vi "Main.vi"(11 "Module Admin":refnum<class "Delacor_lib_QMH_Module Admin.lvclass">) -> ()   [LabVIEW 2020, in "GetTemperature.lvlib"]
doc: "This template is based off of the Queued Message Handler design pattern and the Queued Message Handler project template that ships with LabVIEW.\n\nThe main difference is that the queue is private to this module and communication between modules is performed via Broadcast and Request events.\n\nRequest events are wrapped in public API methods and are handled in the Event Handling Loop (EHL) of this VI. Any module can register for Broadcast events sent by this module. The EHL generates messages based on user interface actions.\n\nThe Message Handling Loop (MHL) processes messages generated by the EHL, or by other messages. The messages are string values, so new messages can be added easily to the Message Cases case structure in the MHL. Each message cluster can also provide an optional value for Message Data, which is a variant that can be converted to whatever message-specific data is required.\n_____\nBased on Delacor QMH Project Template 4.0.0.47.\n_____\nBased on Delacor QMH Project Template 5.0.0.82."
uses:
  GetTemperature.lvlib
  <vilib>/Delacor/Delacor QMH/Libraries/Module Admin_class/Delacor_lib_QMH_Module Admin.lvclass
  Module Data--cluster.ctl
  Stop Argument--cluster.ctl
  <vilib>/Delacor/Delacor QMH/Libraries/Message Queue_class/Delacor_lib_QMH_Message Queue.lvclass/Delacor_lib_QMH_Message Queue.ctl
  <vilib>/Delacor/Delacor QMH/Libraries/Module Admin_class/Delacor_lib_QMH_Module Admin.lvclass/Delacor_lib_QMH_Module Admin.ctl
  Start Acquiring Argument--cluster.ctl
  Start Acquiring (Reply Payload)--cluster.ctl
  Stop Acquiring Argument--cluster.ctl
  Settings Editor/Update Application Settings (Reply Payload)--cluster.ctl
  Settings Editor/Settings--cluster.ctl
  <vilib>/Utility/miscctls.llb/LVPointTypeDef.ctl
  <vilib>/Delacor/Delacor QMH/Libraries/Message Queue_class/Delacor_lib_QMH_Enqueue Message (Single).vi
  <vilib>/Delacor/Delacor QMH/Libraries/Module Admin_class/Delacor_lib_QMH_Get External Launch.vi
  <vilib>/Utility/error.llb/Error Cluster From Error Code.vi
  <vilib>/ErrorRing/Error Ring.xnode
  <vilib>/Delacor/Delacor QMH/Libraries/Message Queue_class/Delacor_lib_QMH_Message Queue.lvclass
  Settings Editor/Settings Editor.lvlib
  Logger/FileLogging.lvlib
panel:
  out "Settings":T1 {"Units" items=["degC", "degF", "kelvin", "raw"]}
  out "Graph Data":waveform(dbl)[](array[waveform])
  out "error out":errorcluster
  # "This is a headless module. Show its panel to confirm that the Settings are updated correctly and other debugging tasks. Use the Settings Editor to change the settings for this module."
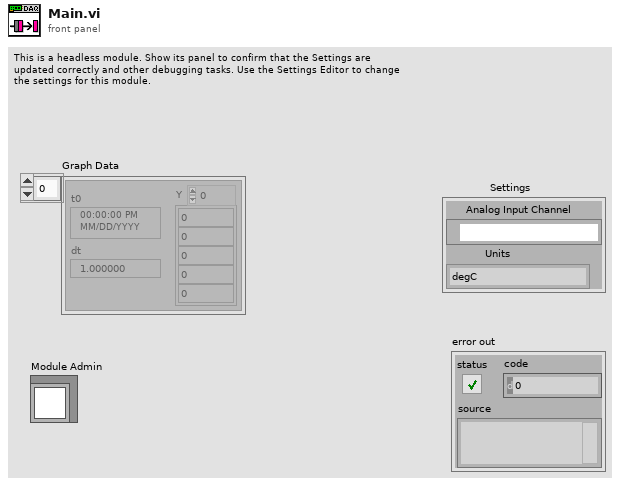
[diagram p1: front panel]
types:
  T1 = typedef "GetTemperature.lvlib/Module Data--cluster.ctl" = cluster{"Analog Input Channel":refnum<k21>, "Units":i32}
  T2 = typedef "Settings Editor.lvlib/Broadcast Events--cluster.ctl" = cluster{"Module Did Init":refnum<user-event>, "Status Updated":refnum<user-event>, "Error Reported":refnum<user-event>, "Module Did Stop":refnum<user-event>, "Update Module Execution Status":refnum<user-event>, "Application Settings Updated":refnum<user-event>}
  T3 = typedef "GetTemperature.lvlib/Request Events--cluster.ctl" = cluster{"Stop Module":refnum<user-event>, "Show Panel":refnum<user-event>, "Hide Panel":refnum<user-event>, "Get Module Execution Status":refnum<user-event>, "Show Diagram":refnum<user-event>, "Stop Acquiring":refnum<user-event>, "Wakeup Helper Loop":refnum<user-event>, "Change Settings":refnum<user-event>, "Calibrate DAQ":refnum<user-event>, "Start Acquiring":refnum<user-event>}
  T4 = enum32{"invalid lock state", "Not Locked", "Locked (No Password)", "Password-protected"}
  T5 = typedef "GetTemperature.lvlib/Stop Argument--cluster.ctl" = cluster{"Origin":string, "Exit via Stop Module Req?":bool, "Wait for Module to stop?":bool}
  T6 = typedef "GetTemperature.lvlib/Start Acquiring Argument--cluster.ctl" = cluster{"Wait Notifier":refnum<notifier>, "wait for reply":bool}
  T7 = typedef "GetTemperature.lvlib/Stop Acquiring Argument--cluster.ctl" = cluster{"Boolean":bool}
  T8 = typedef "Settings Editor.lvlib/Update Application Settings (Reply Payload)--cluster.ctl" = cluster{"Settings":T9, "Update Settings_error":errorcluster}
  T9 = typedef "Settings Editor.lvlib/Settings--cluster.ctl" = cluster{"Log File Base Path":path, "Analog Input Channel":refnum<k21>, "Units":i32}
  T10 = typedef "LVPointTypeDef.ctl" = cluster{"Horizontal":i16, "Vertical":i16}
  T11 = enum32{"Invalid", "Standard", "Closed", "Hidden", "Minimized", "Maximized"}
  T12 = typedef "GetTemperature.lvlib/Start Acquiring (Reply Payload)--cluster.ctl" = cluster{"HW ID":string, "Start Acquiring_error":errorcluster}
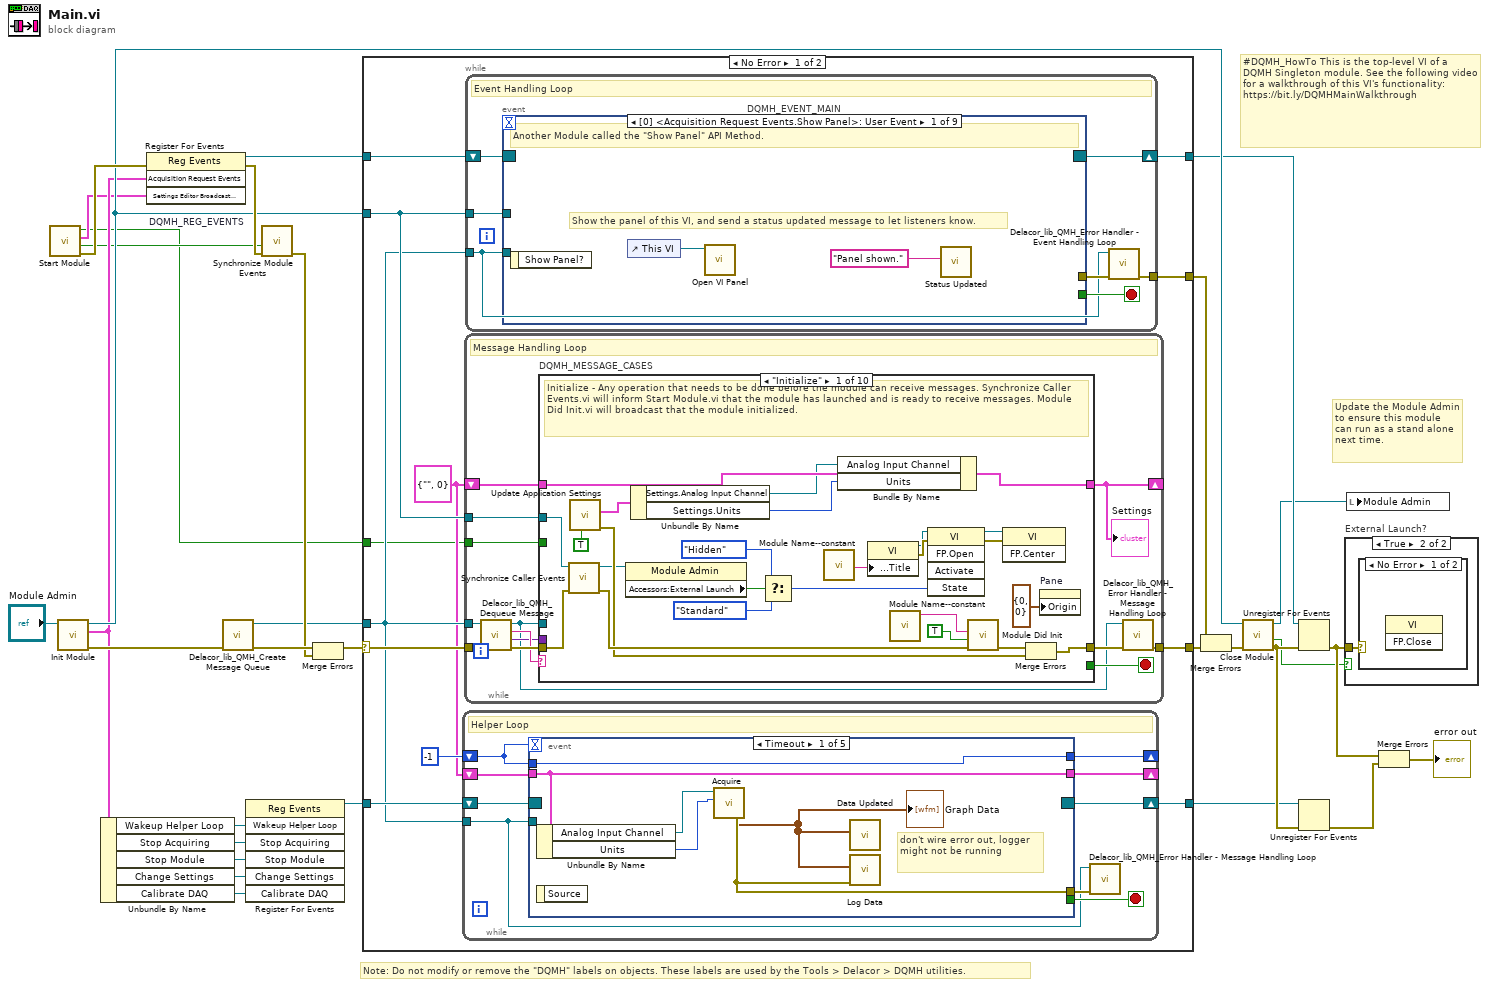
[diagram p0: block diagram]
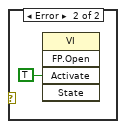
[diagram p3: hidden frame]
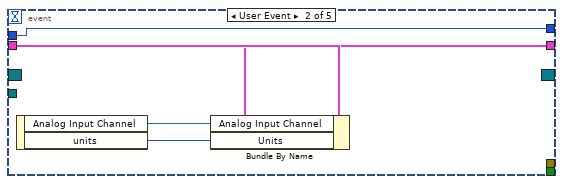
[diagram p4: hidden frame]
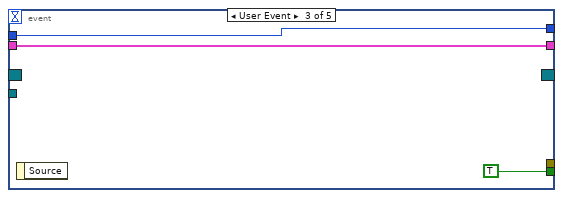
[diagram p5: hidden frame]
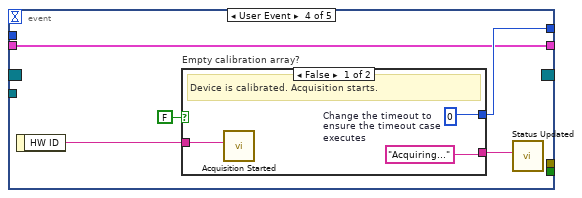
[diagram p6: hidden frame]
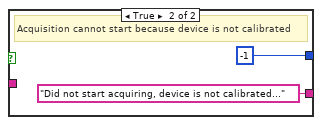
[diagram p7: hidden frame]
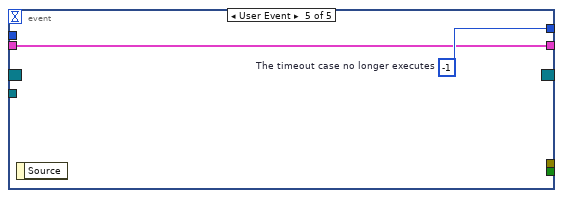
[diagram p8: hidden frame]
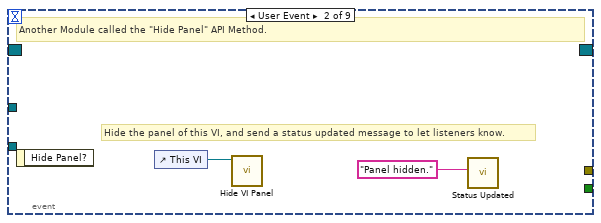
[diagram p9: hidden frame]
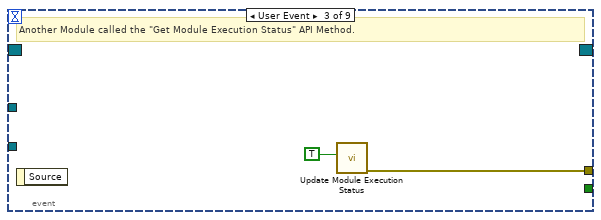
[diagram p10: hidden frame]
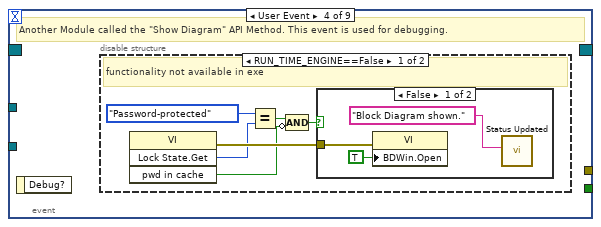
[diagram p11: hidden frame]
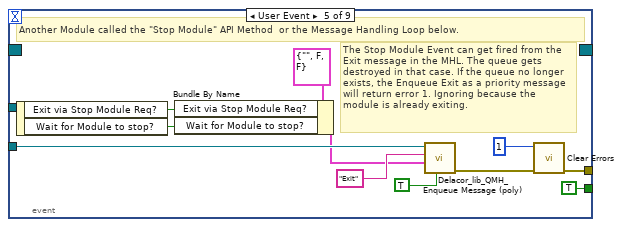
[diagram p14: hidden frame]
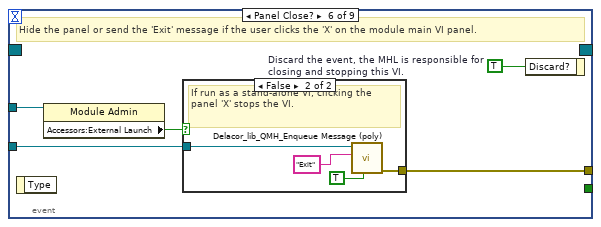
[diagram p15: hidden frame]
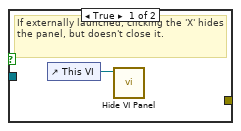
[diagram p16: hidden frame]
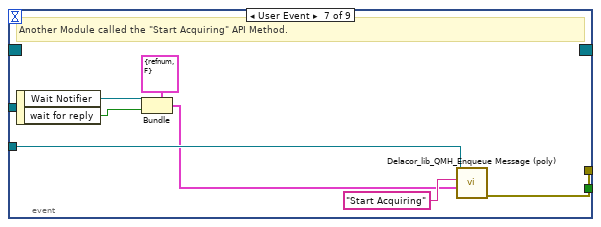
[diagram p17: hidden frame]
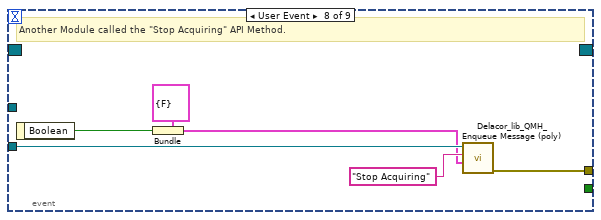
[diagram p18: hidden frame]
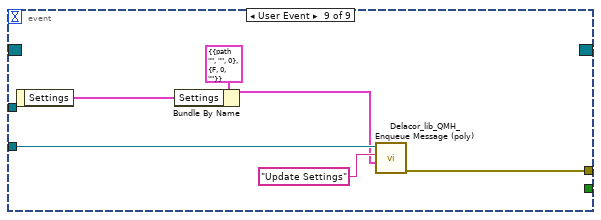
[diagram p19: hidden frame]
diagram:
  # "#DQMH_HowTo This is the top-level VI of a DQMH Singleton module. See the following video for a walkthrough of this VI's functionality: https://bit.ly/DQMHMainWalkthrough"
  # "Note: Do not modify or remove the \"DQMH\" labels on objects. These labels are used by the Tools > Delacor > DQMH utilities."
  # "Update the Module Admin to ensure this module can run as a stand alone next time."
  n1 = call "Start Module.vi"() -> ("error out"=w24:errorcluster, "Wait for Event Sync?"=w5:bool, "Settings Editor Broadcast Events"=w6:T2, "Module Was Already Running?"=w1:bool)  [unwired: 8 in]
  n2 = call "Init Module.vi"("Singleton Module Admin in"="Module Admin") -> ("error out"=w30:errorcluster, "Acquisition Request Events"=w11:T3, "Singleton Module Admin out"=w18:refnum<class "Delacor_lib_QMH_Module Admin.lvclass">)  [unwired: 8 in]
  n3 = Unbundle By Name(w11) -> ("Wakeup Helper Loop"=w7:refnum<user-event>, "Stop Acquiring"=w10:refnum<user-event>, "Stop Module"=w9:refnum<user-event>, "Change Settings"=w4:refnum<user-event>, "Calibrate DAQ"=w3:refnum<user-event>)
  n4 = register-events "DQMH_REG_EVENTS"(error in=w24, w11, w6) -> (reference out=w16:refnum<event-registration>, error out=w23:errorcluster)  [unwired: 1 in]
  n5 = call <vilib>:"Delacor_lib_QMH_Create Message Queue.vi"("error in (no error)"=w30) -> ("error out"=w26:errorcluster, "Message Queue"=w15:refnum<class "Delacor_lib_QMH_Message Queue.lvclass">)  [unwired: 9 in]
  n6 = register-events(w7, w10, w9, w4, w3) -> (reference out=w8:refnum<event-registration>)  [unwired: 2 in, 1 out]
  n7 = call "Synchronize Module Events.vi"("error in (no error)"=w23, "Wait for Event Sync?"=w5) -> ("error out"=w22:errorcluster)  [unwired: 9 in]
  n8 = Merge Errors(w26, w22) -> (w25:errorcluster)
  n9 = case shown="No Error" w25 {
    selector: w25 -> [w41 w274]
    tunnel: [w43 w273] -> w31
    tunnel: [w40 w282] -> w17
    tunnel: w16 -> [w39 w282]
    tunnel: w15 -> [w35 w275]
    tunnel: [w42 _] -> w29
    tunnel: w18 -> [w38 w278]
    tunnel: w8 -> [w36 w277]
    tunnel: [w33 w277] -> w2
    tunnel: w1 -> [w32 w276]
    frame No Error {
      w34 = T1 {"Analog Input Channel"="", "Units"=0} ("Data Cluster")
      n10 = while {
        shift-right: [w51] -> _
        shift-left: -1 -> [w50]
        tunnel: w35 -> [w47]
        shift-right: [w46] -> _
        shift-left: w34 -> [w45]
        shift-right: [w44] -> w33
        shift-left: w36 -> [w49]
        stop <- w48 stop-if-true
        # "Helper Loop"
        n11 = event shown="[0] Timeout" {
          selector: w49 -> [_ _ _ _ _]
          dyn-events: [_ _ _ _ _] -> w44
          timeout: w50 -> [_ _ _ _ _]
          tunnel: [w57 w63 w66 w71 w78] -> w51
          tunnel: w50 -> [w57 w63 w66 _ _]
          tunnel: [_ _ TRUE _ _] -> w48
          tunnel: w47 -> [_ _ _ _ _]
          tunnel: [w58 _ _ _ _] -> w52
          tunnel: [w56 w61 w64 w68 w77] -> w46
          tunnel: w45 -> [w56 w62 w64 w68 w77]
          event Timeout {
            # "don't wire error out, logger might not be running"
            n12 = Unbundle By Name(w56) -> ("Analog Input Channel"=w55:refnum<k21>, "Units"=w53:i32)
            n13 = event-data() -> ()  [unwired: 1 in, 1 out]
            n14 = call "Acquire.vi"("Units"=w53, "physical channels"=w55) -> ("error out"=w58:errorcluster, "Graph Data"=w54:waveform(dbl)[])  [unwired: 8 in]
            "Graph Data" <- w54
            n15 = call "Data Updated.vi"("Graph Data"=w54) -> ()  [unwired: 10 in, 1 out]
            n16 = call "Log Data.vi"("error in (no error)"=w58, "Waveforms"=w54) -> ()  [unwired: 9 in, 1 out]
          }
          event User Event {
            n17 = event-data() -> ("Analog Input Channel"=w60:refnum<k21>, "units"=w59:i32)  [unwired: 1 in]
            n18 = Bundle By Name(cluster=w62, "Analog Input Channel"=w60, "Units"=w59) -> (w61:T1)
          }
          event User Event {
            n19 = event-data() -> ()  [unwired: 1 in, 1 out]
          }
          event User Event {
            n20 = event-data() -> ("HW ID"=w69:string)  [unwired: 1 in]
            n21 = case "Empty calibration array?" shown="False" FALSE {
              tunnel: ["Acquiring..." ("Status") "Did not start acquiring, device is not calibrated..." ("Status")] -> w70
              tunnel: [w73 -1] -> w71
              tunnel: w69 -> [w74 _]
              frame False {
                w73 = 0  # Change the timeout to ensure the timeout case executes
                # "Device is calibrated. Acquisition starts."
                n22 = call "Acquisition Started.vi"("HW ID"=w74) -> ()  [unwired: 10 in, 1 out]
              }
              frame True {
                # "Acquisition cannot start because device is not calibrated"
              }
            }
            n23 = call "Status Updated.vi"("Status"=w70) -> ()  [unwired: 10 in, 1 out]
          }
          event User Event {
            w78 = -1  # The timeout case no longer executes
            n24 = event-data() -> ()  [unwired: 1 in, 1 out]
          }
        }
        n25 = call-dynamic "Delacor_lib_QMH_Error Handler - Message Handling Loop.vi"("error in (no error)"=w52, "Message Queue in"=w47) -> ()  [unwired: 8 in, 2 out]
      }
      n26 = while {
        tunnel: w35 -> [w145]
        shift-right: [w141] -> _
        shift-left: w34 -> [w149]
        tunnel: w41 -> [w152]
        tunnel: [w150] -> w43
        tunnel: w38 -> [w143]
        tunnel: w32 -> [w142]
        stop <- w148 stop-if-true
        # "Message Handling Loop"
        n27 = call-dynamic "Delacor_lib_QMH_Dequeue Message.vi"("error in (no error)"=w152, "Message Queue in"=w145) -> ("error out"=w151:errorcluster, "Message Data"=w146:variant, "Message"=w147:string, "Message Queue out"=w144:refnum<class "Delacor_lib_QMH_Message Queue.lvclass">)  [unwired: 6 in]
        n28 = case "DQMH_MESSAGE_CASES" shown="\"Initialize\"" w147 {
          selector: w147 -> [_ _ _ _ _ _ _ _ _ w260]
          tunnel: w144 -> [_ _ _ _ _ _ _ w225 w249 _]
          tunnel: w151 -> [w176 w180 w193 w207 w216 w219 w221 w232 w256 w263]
          tunnel: [w173 w180 w191 w205 w210 w218 w221 w228 w253 w264] -> w153
          tunnel: w149 -> [w163 w179 w181 w202 w213 w217 w220 w227 w241 w261]
          tunnel: [w158 w179 w189 w202 w213 w217 w220 w227 w241 w261] -> w141
          tunnel: [_ _ _ _ _ _ _ _ w248 _] -> w148
          tunnel: w146 -> [_ _ w188 w204 w214 _ _ w226 w247 _]
          tunnel: w143 -> [w164 _ _ _ _ _ _ w224 w242 _]
          tunnel: w142 -> [_ _ _ _ _ _ _ _ w239 _]
          frame "Initialize" {
            # "Initialize - Any operation that needs to be done before the module can receive messages. Synchronize Caller Events.vi will inform Start Module.vi that the module has launched and is ready to receive messages. Module Did Init.vi will broadcast that the module initialized."
            n29 = call "Synchronize Caller Events.vi"("error in (no error)"=w176, "Singleton Module Admin in"=w164) -> ("error out"=w175:errorcluster, "Singleton Module Admin out"=w160:refnum<class "Delacor_lib_QMH_Module Admin.lvclass">)  [unwired: 8 in]
            n30 = call "Update Application Settings.vi"("wait for reply (T)"=TRUE) -> ("error out"=w172:errorcluster, "Reply Payload"=w157:T8)  [unwired: 8 in, 1 out]
            n31 = property class="Module Admin"(reference=w160) -> ("Accessors:External Launch"=w168:bool)  [unwired: 1 in, 2 out]
            n32 = Unbundle By Name(w157) -> ("Settings.Analog Input Channel"=w155:refnum<k21>, "Settings.Units"=w154:i32)
            n33 = Select(t=T11."Hidden" ("State"), s=w168, f=T11."Standard" ("State")) -> (s? t:f=w165:T11)
            n34 = call "Module Name--constant.vi"() -> ("Module Name"=w171:string)  [unwired: 11 in]
            n35 = Bundle By Name(cluster=w163, "Analog Input Channel"=w155, "Units"=w154) -> (w158:T1)
            n36 = property class="VI"("Front Panel.Title"=w171) -> (reference out=w170:refnum<vi>, error out=w178:errorcluster)  [unwired: 2 in]
            n37 = call "Module Name--constant.vi"() -> ("Module Name"=w161:string)  [unwired: 11 in]
            n38 = invoke class="VI" method="FP.Open"(reference=w170, error in=w178, "State"=w165) -> (reference out=w169:refnum<vi>, error out=w177:errorcluster)  [unwired: 2 in, 3 out]
            n39 = call "Module Did Init.vi"("error in (no error)"=w175, "Initialized?"=TRUE, "Origin"=w161) -> ("error out"=w174:errorcluster)  [unwired: 8 in]
            n40 = invoke class="VI" method="FP.Center"(reference=w169, error in=w177) -> ()  [unwired: 1 in, 3 out]
            n41 = Merge Errors(w174, w172) -> (w173:errorcluster)
            n42 = property on="Pane" class="Pane"("Origin"=T10 {"Horizontal"=0, "Vertical"=0}) -> ()  [unwired: 2 in, 2 out]
          }
          frame "--- Module Specific ---" {
            # "Separator -- The following cases handle messages specific to this Module."
          }
          frame "Start Acquiring" {
            # "Requests Acquisition Module to start acquiring."
            n43 = Variant To Data(error in=w193, type=T6 {"Wait Notifier"=refnum, "wait for reply"=FALSE} ("Start Acquisition Argument"), Variant=w188) -> (data=w186:T6, error out=w190:errorcluster)
            n44 = in-place {
              in-place-border: [w199] -> w192
              in-place-border: w190 -> [w198]
              in-place-border: [w194] -> w182
              n45 = in-place-cluster #1(w181) -> ("Analog Input Channel"=w195:refnum<k21>)
              n46 = call "Initialize Hardware References.vi"("error in (no error)"=w198, "HW Refnum in"=w195) -> ("error out"=w197:errorcluster, "HW Refnum out"=w196:string)  [unwired: 8 in]
              n47 = call "Configure Hardware.vi"("error in (no error)"=w197, "HW Refnum in"=w196) -> ("error out"=w199:errorcluster, "HW Refnum out"=w194:string)  [unwired: 8 in]
              n48 = in-place-cluster #1("Analog Input Channel"=w194) -> (w189:T1)
            }
            n49 = Bundle By Name(cluster=T12 {"HW ID"="", "Start Acquiring_error"={"status"=FALSE, "code"=0, "source"=""}} ("Start Acquisition (Reply Payload)"), "HW ID"=w182, "Start Acquiring_error"=w192) -> (w184:T12)
            n50 = Unbundle By Name(w186) -> ("Wait Notifier"=w185:refnum<notifier>)
            n51 = call "Wakeup Helper Loop.vi"("error in (no error)"=w192, "HW ID"=w182) -> ("error out"=w191:errorcluster)  [unwired: 9 in]
            n52 = Send Notification(notification=w184, notifier=w185) -> ()  [unwired: 1 in, 2 out]
          }
          frame "Stop Acquiring" {
            # "Requests the Acquisition Module to stop acquiring"
            n53 = Variant To Data(error in=w207, type=T7 {"Boolean"=FALSE} ("Stop Acquiring Argument"), Variant=w204) -> (error out=w206:errorcluster)  [unwired: 1 out]
            n54 = Unbundle By Name(w202) -> ("Analog Input Channel"=w201:refnum<k21>)
            n55 = call "Stop Acquisition.vi"("error in (no error)"=w206, "HW Refnum"=w201) -> ("error out"=w205:errorcluster)  [unwired: 9 in]
            n56 = call "Acquisition Stopped.vi"("error in (no error)"=w205) -> ()  [unwired: 10 in, 1 out]
            n57 = call "Status Updated.vi"("error in (no error)"=w205, "Status"="Acquisition Stopped") -> ()  [unwired: 9 in, 1 out]
          }
          frame "Update Settings" {
            # "Send the Change Settings event to the helper loop."
            # "The Settings Editor broadcasted that the settings have changed."
            n58 = Variant To Data(error in=w216, type=T8 {"Settings"={"Log File Base Path"=path "", "Analog Input Channel"="", "Units"=0}, "Update Settings_error"={"status"=FALSE, "code"=0, "source"=""}} ("Settings Updated Argument"), Variant=w214) -> (data=w211:T8, error out=w215:errorcluster)
            n59 = Unbundle By Name(w211) -> ("Settings.Analog Input Channel"=w208:refnum<k21>)  [unwired: 1 out]
            n60 = call "Change Settings.vi"("error in (no error)"=w215, "Analog Input Channel"=w208) -> ("error out"=w210:errorcluster)  [unwired: 9 in]
            n61 = call "Status Updated.vi"("error in (no error)"=w210, "Status"="Settings Updated") -> ()  [unwired: 9 in, 1 out]
          }
          frame "---Copy This Frame---" {
            # "Duplicate this frame when creating new messages.  Change this comment in the duplicated frame to describe this message."
            n62 = Merge Errors(w219) -> (w218:errorcluster)
          }
          frame "--- Exit and Error Handling---" {
            # "Separator - The following cases handle errors and exit messages."
          }
          frame "Error" {
            # "Error - Check the error message data and respond accordingly. This message is sent by the \"Error Handler\" VIs at the end of each loop in this application."
            n63 = property class="Module Admin"(reference=w224) -> ("Accessors:External Launch"=w223:bool)  [unwired: 1 in, 2 out]
            n64 = Variant To Data(error in=w232, type=errorcluster {"status"=FALSE, "code"=0, "source"=""} ("error constant"), Variant=w226) -> (data=w233:errorcluster, error out=w230:errorcluster)
            n65 = call "Module Name--constant.vi"() -> ("Module Name"=w222:string)  [unwired: 11 in]
            n66 = call "Error Reported.vi"("Additional Information"=w222, "Error"=w233) -> ()  [unwired: 9 in, 1 out]
            n67 = case shown="False" w223 {
              tunnel: [w238 _] -> w229
              tunnel: w225 -> [w236 _]
              tunnel: w233 -> [w237 _]
              frame False {
                # "If the module is running standalone, then pop up an error dialog and call the \"Exit\" message."
                n68 = call <vilib>:"Simple Error Handler.vi"("error in (no error)"=w237) -> ()  [unwired: 4 in, 5 out]
                n69 = call-poly <vilib>:"Delacor_lib_QMH_Enqueue Message (poly).vi"("Priority Message? (F)"=TRUE, "Message"="Exit", "Message Queue in"=w236) -> ("error out"=w238:errorcluster)  [unwired: 7 in, 1 out]
              }
              frame True {
                # "If the module was launched externally, calling the Error Reported broadcast VI is the only action performed by the \"Error\" message. The module's caller can then process the error appropriately."
              }
            }
            n70 = Merge Errors(w230, w229) -> (w228:errorcluster)
            n71 = local write "error out"(w228) -> ()
          }
          frame "Exit" {
            w246 = 91  # 91: not all Exit messages will have an argument
            w248 = TRUE  # Stop the VI
            # "Release the message queue reference"
            # "Exit - Exit the application."
            n72 = Variant To Data(error in=w256, type=T5 {"Origin"="", "Exit via Stop Module Req?"=FALSE, "Wait for Module to stop?"=FALSE} ("Stop Argument"), Variant=w247) -> (data=w244:T5, error out=w252:errorcluster)
            n73 = call <vilib>:"Clear Errors.vi"("error in (no error)"=w252, "specific error code to clear (0: all)"=w246) -> ("error out"=w255:errorcluster)  [unwired: 4 in, 1 out]
            n74 = Unbundle By Name(w241) -> ("Analog Input Channel"=w240:refnum<k21>)
            n75 = control-ref of="This VI"() -> (w243:refnum<vi>)
            n76 = call "Handle Exit.vi"("Stop Argument"=w244, "Admin in"=w242, "VI reference"=w243) -> ("error out"=w251:errorcluster)  [unwired: 7 in, 1 out]
            n77 = call "Close Hardware References.vi"("HW Refnum in"=w240) -> ("error out"=w250:errorcluster)  [unwired: 9 in, 1 out]
            n78 = call-dynamic "Delacor_lib_QMH_Release Message Queue.vi"("error in (no error)"=w255, "Message Queue"=w249) -> ("error out"=w254:errorcluster)  [unwired: 9 in]
            n79 = case "Settings Editor was\nalready running?" shown="False" w239 {
              frame False {
                n80 = call "Module Name--constant.vi"() -> ("Module Name"=w258:string)  [unwired: 11 in]
                n81 = call "Stop Module.vi"("Wait for Module to Stop? (F)"=TRUE, "Origin"=w258) -> ()  [unwired: 9 in, 1 out]
              }
              frame True {
                # "Another Module is\nin charge of stopping Settings Editor"
              }
            }
            n82 = Merge Errors(w254, w251, w250) -> (w253:errorcluster)
          }
          frame Default {
            # "'Default' case only runs if there is a message that isn't defined in any of the other cases.  Output a programming error."
            n83 = call "Module Name--constant.vi"() -> ("Module Name"=w259:string)  [unwired: 11 in]
            n84 = xnode "Error Ring"("parameter 0"=w260, "parameter 1"=w259) -> ("error out"=w262:errorcluster)
            n85 = Merge Errors(w263, w262) -> (w264:errorcluster)
          }
        }
        "Settings" <- w141
        n86 = call-dynamic "Delacor_lib_QMH_Error Handler - Message Handling Loop.vi"("error in (no error)"=w153, "Message Queue in"=w144) -> ("dup error in"=w150:errorcluster)  [unwired: 8 in, 1 out]
      }
      n87 = while {
        tunnel: w35 -> [w79]
        shift-right: [w82] -> w40
        shift-left: w39 -> [w83]
        tunnel: [w84] -> w42
        tunnel: w38 -> [w80]
        stop <- w81 stop-if-true
        # "Event Handling Loop"
        n88 = event "DQMH_EVENT_MAIN" shown="[0] <Acquisition Request Events.Show Panel>: User Event" {
          selector: w83 -> [_ _ _ _ _ _ _ _ _]
          dyn-events: [_ _ _ _ _ _ _ _ _] -> w82
          timeout: _ -> [_ _ _ _ _ _ _ _ _]
          tunnel: [_ _ _ _ TRUE ("Discard?") _ _ _ _] -> w81
          tunnel: w79 -> [_ _ _ _ w107 w114 w128 w133 w138]
          tunnel: [_ _ w91 _ w110 w116 w124 w134 w140] -> w85
          tunnel: w80 -> [_ _ _ _ _ w113 _ _ _]
          event User Event {
            # "Show the panel of this VI, and send a status updated message to let listeners know."
            # "Another Module called the \"Show Panel\" API Method."
            n89 = event-data() -> ()  [unwired: 1 in, 1 out]
            n90 = control-ref of="This VI"() -> (w87:refnum<vi>)
            n91 = call "Open VI Panel.vi"("VI"=w87) -> ()  [unwired: 10 in, 1 out]
            n92 = call "Status Updated.vi"("Status"="Panel shown." ("format string")) -> ()  [unwired: 10 in, 1 out]
          }
          event User Event {
            # "Hide the panel of this VI, and send a status updated message to let listeners know."
            # "Another Module called the \"Hide Panel\" API Method."
            n93 = event-data() -> ()  [unwired: 1 in, 1 out]
            n94 = control-ref of="This VI"() -> (w89:refnum<vi>)
            n95 = call "Hide VI Panel.vi"("VI"=w89) -> ()  [unwired: 10 in, 1 out]
            n96 = call "Status Updated.vi"("Status"="Panel hidden." ("format string")) -> ()  [unwired: 10 in, 1 out]
          }
          event User Event {
            # "Another Module called the \"Get Module Execution Status\" API Method."
            n97 = event-data() -> ()  [unwired: 1 in, 1 out]
            n98 = call "Update Module Execution Status.vi"("Running?"=TRUE) -> ("error out"=w91:errorcluster)  [unwired: 10 in]
          }
          event User Event {
            # "Another Module called the \"Show Diagram\" API Method. This event is used for debugging."
            n99 = event-data() -> ()  [unwired: 1 in, 1 out]
            n100 = disable-structure shown="RUN_TIME_ENGINE==False" {
              frame condition #0 (active) {
                # "functionality not available in exe"
                n101 = invoke class="VI" method="Lock State.Get"() -> (error out=w97:errorcluster, "Get Lock State"=w96:T4, "pwd in cache"=w93:bool)  [unwired: 4 in, 1 out]
                n102 = Equal?(x=T4."Password-protected", y=w96) -> (x = y?=w94:bool)
                n103 = Compound Arithmetic op=AND(w94, invert w93) -> (w92:bool)
                n104 = case shown="False" w92 {
                  tunnel: w97 -> [w100 _]
                  frame False {
                    n105 = property class="VI"(error in=w100, "BDWin.Open"=TRUE ("Block Diagram Window:Open")) -> ()  [unwired: 1 in, 2 out]
                    n106 = call "Status Updated.vi"("Status"="Block Diagram shown." ("format string")) -> ()  [unwired: 10 in, 1 out]
                  }
                  frame True {
                    # "Password-protected VI, and the password is not in the cache. Do not show the diagram."
                  }
                }
              }
              frame condition #1 {
              }
            }
          }
          event User Event {
            # "The Stop Module Event can get fired from the Exit message in the MHL. The queue gets destroyed in that case. If the queue no longer exists, the Enqueue Exit as a priority message will return error 1. Ignoring because the module is already exiting."
            # "Another Module called the \"Stop Module\" API Method  or the Message Handling Loop below."
            n107 = event-data() -> ("Exit via Stop Module Req?"=w103:bool, "Wait for Module to stop?"=w102:bool)  [unwired: 1 in]
            n108 = Bundle By Name(cluster=T5 {"Origin"="", "Exit via Stop Module Req?"=FALSE, "Wait for Module to stop?"=FALSE} ("Stop Argument"), "Exit via Stop Module Req?"=w103, "Wait for Module to stop?"=w102) -> (w101:T5)
            n109 = call-poly <vilib>:"Delacor_lib_QMH_Enqueue Message (poly).vi"("Priority Message? (F)"=TRUE, "Message Data"=w101, "Message"="Exit", "Message Queue in"=w107) -> ("error out"=w111:errorcluster)  [unwired: 6 in, 1 out]
            n110 = call <vilib>:"Clear Errors.vi"("error in (no error)"=w111, "specific error code to clear (0: all)"=1) -> ("error out"=w110:errorcluster)  [unwired: 4 in, 1 out]
          }
          event Panel Close? {
            w115 = TRUE  # Discard the event, the MHL is responsible for closing and stopping this VI.
            # "Hide the panel or send the 'Exit' message if the user clicks the 'X' on the module main VI panel."
            n111 = event-data() -> ()  [unwired: 1 in, 1 out]
            n112 = property class="Module Admin"(reference=w113) -> ("Accessors:External Launch"=w112:bool)  [unwired: 1 in, 2 out]
            n113 = case shown="False" w112 {
              tunnel: w114 -> [_ w120]
              tunnel: [_ w121] -> w116
              frame True {
                # "If externally launched, clicking the 'X' hides the panel, but doesn't close it."
                n114 = control-ref of="This VI"() -> (w117:refnum<vi>)
                n115 = call "Hide VI Panel.vi"("VI"=w117) -> ()  [unwired: 10 in, 1 out]
              }
              frame False {
                # "If run as a stand-alone VI, clicking the panel 'X' stops the VI."
                n116 = call-poly <vilib>:"Delacor_lib_QMH_Enqueue Message (poly).vi"("Priority Message? (F)"=TRUE, "Message"="Exit", "Message Queue in"=w120) -> ("error out"=w121:errorcluster)  [unwired: 7 in, 1 out]
              }
            }
            n117 = event-data("Discard?"=w115) -> ()  [unwired: 1 in, 1 out]
          }
          event User Event {
            # "Another Module called the \"Start Acquiring\" API Method."
            n118 = event-data() -> ("Wait Notifier"=w123:refnum<notifier>, "wait for reply"=w122:bool)  [unwired: 1 in]
            n119 = Bundle(cluster=T6 {"Wait Notifier"=refnum, "wait for reply"=FALSE} ("Start Acquisition Argument"), "Wait Notifier"=w123, "wait for reply"=w122) -> (w125:T6)
            n120 = call-poly <vilib>:"Delacor_lib_QMH_Enqueue Message (poly).vi"("Message Data"=w125, "Message"="Start Acquiring", "Message Queue in"=w128) -> ("error out"=w124:errorcluster)  [unwired: 7 in, 1 out]
          }
          event User Event {
            # "Another Module called the \"Stop Acquiring\" API Method."
            n121 = event-data() -> ("Boolean"=w129:bool)  [unwired: 1 in]
            n122 = Bundle(cluster=T7 {"Boolean"=FALSE} ("Stop Acquiring Argument"), "Boolean"=w129) -> (w130:T7)
            n123 = call-poly <vilib>:"Delacor_lib_QMH_Enqueue Message (poly).vi"("Message Data"=w130, "Message"="Stop Acquiring", "Message Queue in"=w133) -> ("error out"=w134:errorcluster)  [unwired: 7 in, 1 out]
          }
          event User Event {
            n124 = event-data() -> ("Settings"=w135:T9)  [unwired: 1 in]
            n125 = Bundle By Name(cluster=T8 {"Settings"={"Log File Base Path"=path "", "Analog Input Channel"="", "Units"=0}, "Update Settings_error"={"status"=FALSE, "code"=0, "source"=""}} ("Settings Updated Argument"), "Settings"=w135) -> (w137:T8)
            n126 = call-poly <vilib>:"Delacor_lib_QMH_Enqueue Message (poly).vi"("Message Data"=w137, "Message"="Update Settings", "Message Queue in"=w138) -> ("error out"=w140:errorcluster)  [unwired: 7 in, 1 out]
          }
        }
        n127 = call-dynamic "Delacor_lib_QMH_Error Handler - Event Handling Loop.vi"("error in (no error)"=w85, "Message Queue in"=w79) -> ("dup error in"=w84:errorcluster)  [unwired: 8 in, 1 out]
      }
    }
    frame Error {
      # "Synchronize Caller Events.vi will inform Start Module.vi that the module has launched and will let the code calling Start Module.vi register for broadcasts and would permit the caller receive the broadcast that an error occurred at launch time."
      n128 = call "Synchronize Caller Events.vi"("Singleton Module Admin in"=w278) -> ("error out"=w283:errorcluster)  [unwired: 9 in, 1 out]
      n129 = call-dynamic "Delacor_lib_QMH_Release Message Queue.vi"("error in (no error)"=w274, "Message Queue"=w275) -> ("error out"=w273:errorcluster)  [unwired: 9 in]
      n130 = call "Module Name--constant.vi"() -> ("Module Name"=w281:string)  [unwired: 11 in]
      n131 = case "Settings Editor was\nalready running?" shown="False" w276 {
        frame False {
          n132 = call "Module Name--constant.vi"() -> ("Module Name"=w286:string)  [unwired: 11 in]
          n133 = call "Stop Module.vi"("Wait for Module to Stop? (F)"=TRUE, "Origin"=w286) -> ()  [unwired: 9 in, 1 out]
        }
        frame True {
          # "Another Module is\nin charge of stopping Settings Editor"
        }
      }
      n134 = Format Into String(format string="An error occurred during initialization. %s is no longer running.", w281) -> (resulting string=w279:string)  [unwired: 2 in, 1 out]
      n135 = Merge Errors(w273, w283) -> (w284:errorcluster)
      n136 = call "Error Reported.vi"("Additional Information"=w279, "Error"=w284) -> ()  [unwired: 9 in, 1 out]
    }
  }
  n137 = Merge Errors(w29, w31) -> (w28:errorcluster)
  n138 = call "Close Module.vi"("error in (no error)"=w28, "Module Admin in"=w18) -> ("error out"=w21:errorcluster, "External Launch"=w12:bool, "Module Admin out"=w13:refnum<class "Delacor_lib_QMH_Module Admin.lvclass">)  [unwired: 7 in]
  n139 = Unregister For Events(event registration refnum=w17, error in=w21) -> (error out=w27:errorcluster)
  n140 = Unregister For Events(event registration refnum=w2, error in=w21) -> (error out=w19:errorcluster)
  n141 = case "External Launch?" shown="True" w12 {
    tunnel: w27 -> [_ w287]
    frame False {
    }
    frame True {
      n142 = case shown="No Error" w287 {
        frame No Error {
          n143 = invoke class="VI" method="FP.Close"() -> ()  [unwired: 3 in, 3 out]
        }
        frame Error {
          n144 = invoke class="VI" method="FP.Open"("Activate"=TRUE ("Activate?")) -> ()  [unwired: 4 in, 5 out]
        }
      }
    }
  }
  n145 = local write "Module Admin"(w13) -> ()
  n146 = Merge Errors(w27, w19) -> (→"error out":errorcluster)
